vi "Fix Duplicates in Tree.vi"(8 "error in (no error)":errorcluster, 11 "Data in":T1) -> (0 "error out":errorcluster, 3 "Data out":T1)   [LabVIEW 2020, in "Peek Window.lvlib"]
uses:
  Peek Window.lvlib
  MHL Data Cluster.ctl
  Open Diagram Argument--cluster.ctl
  VI Types Enum.ctl
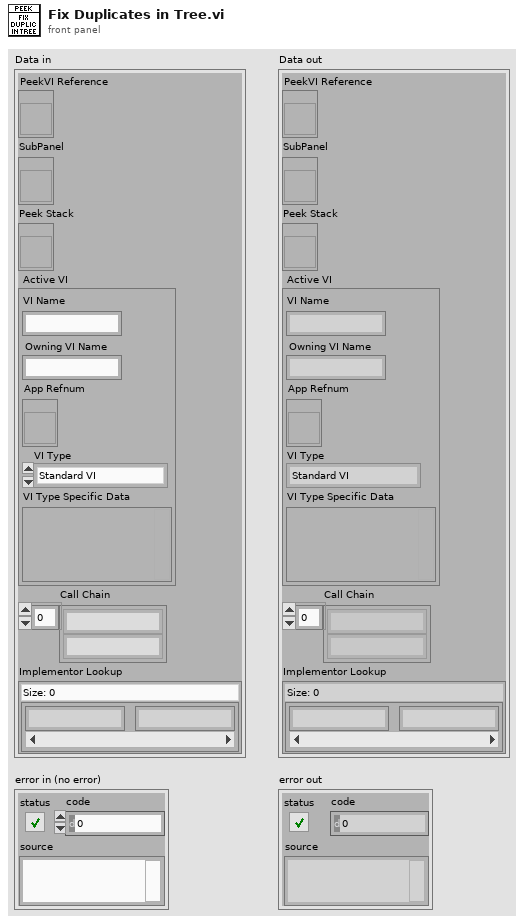
[diagram p1: front panel]
types:
  T1 = typedef "Peek Window.lvlib/MHL Data Cluster.ctl" = cluster{"PeekVI Reference":refnum<vi>, "SubPanel":refnum<vi>, "Peek Stack":refnum<vi>, "Active VI":T2, "Call Chain":string[], "Implementor Lookup":map{string, string}}
  T2 = typedef "Peek Window.lvlib/Open Diagram Argument--cluster.ctl" = cluster{"VI Name":string, "Owning VI Name":string, "App Refnum":refnum<vi>, "VI Type":T3, "VI Type Specific Data":variant}
  T3 = typedef "Peek Window.lvlib/VI Types Enum.ctl" = enum16{"Standard VI", "Dynamic Dispatch VI", "Malleable VI", "Express VI", "Polymorphic VI", "Missing VI"}
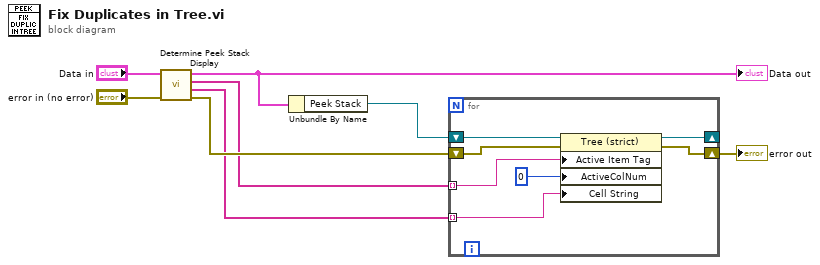
[diagram p0: block diagram]
diagram:
  n1 = call "Determine Peek Stack Display.vi"("error in"="error in (no error)", "Module Data"="Data in") -> ("error out"=w3:errorcluster, "Unique VI Names for Display"=w2:string[], "Tags"=w1:string[], "Module Data"=w5:T1)  [unwired: 6 in]
  "Data out" <- w5
  n2 = Unbundle By Name(w5) -> ("Peek Stack"=w7:refnum<vi>)
  n3 = for {
    shift-right: [w13] -> _
    shift-left: w7 -> [w15]
    tunnel: w1 -> [w12] mode=indexing
    tunnel: w2 -> [w10] mode=indexing
    shift-right: [w9] -> w8
    shift-left: w3 -> [w14]
    n4 = property class="Tree (strict)"(reference=w15, error in=w14, "Active Item Tag"=w12, "ActiveColNum"=0, "Cell String"=w10) -> (reference out=w13:refnum<vi>, error out=w9:errorcluster)
  }
  "error out" <- w8
